vi "2 Runprotect.vi"(10 "Wind Records":dbl[][](array[numeric])) -> ()   [LabVIEW 2011]
doc: "This VI is launched, when the Runprotect Boolean in the Wind Records VI is activated.\nIt calculates a Wind Direction and a Windspeed out of the REcords that were taken before.\nIn this calculations, the newer values are counted higher than older values.\nThe calculated values are absolute values and we use the VI \"1 Wind Calculator\" from the Simulation Platform to calculate the Apparent Wind."
uses:
  2 Globals/2 Global.vi
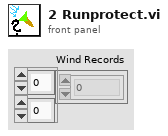
[diagram p1: front panel]
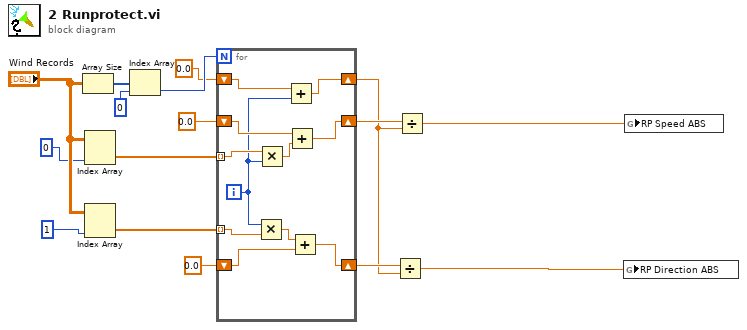
[diagram p0: block diagram]
diagram:
  n1 = Array Size(array="Wind Records") -> (size(s)=w15:i32[])
  n2 = Index Array(array="Wind Records", index (col)=0) -> (element=w13:dbl[])  [unwired: 1 in]
  n3 = Index Array(array="Wind Records", index (col)=1) -> (element=w12:dbl[])  [unwired: 1 in]
  n4 = Index Array(array=w15, index=0) -> (element=w14:i32)
  n5 = for {
    N: w14 -> [_]
    tunnel: w13 -> [w27] mode=indexing
    tunnel: w12 -> [w26] mode=indexing
    shift-right: [w20] -> w9
    shift-left: 0.0 -> [w25]
    shift-right: [w21] -> w8
    shift-left: 0.0 -> [w22]
    shift-right: [w17] -> w1
    shift-left: 0.0 -> [w19]
    i -> [w18]
    n6 = Multiply(x=w18, y=w26) -> (x*y=w23:dbl)
    n7 = Multiply(x=w27, y=w18) -> (x*y=w24:dbl)
    n8 = Add(x=w19, y=w18) -> (x+y=w17:dbl)
    n9 = Add(x=w25, y=w24) -> (x+y=w20:dbl)
    n10 = Add(x=w23, y=w22) -> (x+y=w21:dbl)
  }
  n11 = Divide(x=w8, y=w1) -> (x/y=w5:dbl)
  n12 = Divide(x=w9, y=w1) -> (x/y=w6:dbl)
  n13 = global write "2 Global.vi" "RP Direction ABS"(w5) -> ()
  n14 = global write "2 Global.vi" "RP Speed ABS"(w6) -> ()
